vi "RichToFlatniswitch_grpc_GetNextInterchangeWarningResponse.vi"(5 "OutputClusterType":T1, 11 "InputCluster":T2) -> (3 "OutputCluster":T1)   [LabVIEW 2021, in "NI Switch_client.lvlib"]
uses:
  NI Switch_client.lvlib
  niswitch_grpc_GetNextInterchangeWarningResponse_Flat.ctl
  niswitch_grpc_GetNextInterchangeWarningResponse.ctl
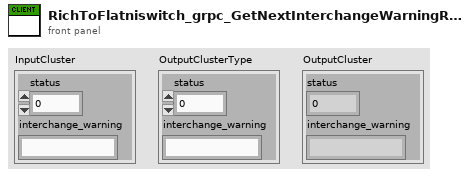
[diagram p1: front panel]
types:
  T1 = typedef "NI Switch_client.lvlib/niswitch_grpc_GetNextInterchangeWarningResponse_Flat.ctl" = cluster{"status":i32, "interchange_warning":string}
  T2 = typedef "NI Switch_client.lvlib/niswitch_grpc_GetNextInterchangeWarningResponse.ctl" = cluster{"status":i32, "interchange_warning":string}
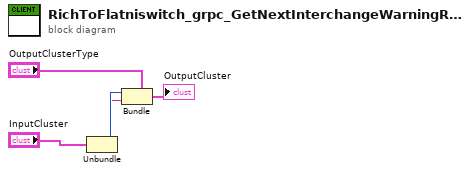
[diagram p0: block diagram]
diagram:
  n1 = Unbundle "Unbundle"("InputCluster") -> ("status"=w2:i32, "interchange_warning"=w1:string)
  n2 = Bundle "Bundle"(cluster="OutputClusterType", "status"=w2, "interchange_warning"=w1) -> (→"OutputCluster":T1)
